vi "Configure Multi Eval Meas Limit Emission Mask Test Tolerance.vi"(7 "Tolerance 30-40 (3.46)":dbl=3.46 format="%^.3e", 8 "error in (no error)":errorcluster, 9 "Tolerance 23-30 (3.21)":dbl=3.21 format="%^.3e", 10 "Instance (1)":T1=1, 11 "VISA resource name":refnum<visa-resource-name>) -> (0 "error out":errorcluster, 3 "VISA resource name out":refnum<visa-resource-name>)   [LabVIEW 2015, in "Rohde&Schwarz CMXP NR FR2 Measurement.lvlib"]
doc: "Defines the test tolerance for spectrum emission masks, depending on the carrier frequency.\n\nAttribute:\nRSCMXPNRFR2M_ATTR_MULTI_EVAL_MEASUREMENT_LIMIT_EMISSION_MASK_TEST_TOLERANCE\n\nRemote-control command:\nCONFigure:NRMMw:MEAS<i>:MEValuation:LIMit:SEMask:ATTolerance"
uses:
  <instrlib>/Rohde&Schwarz CMXP NR FR2 Measurement/Rohde&Schwarz CMXP NR FR2 Measurement.lvlib
  <instrlib>/Rohde&Schwarz CMXP NR FR2 Measurement/Private/_Instance.ctl
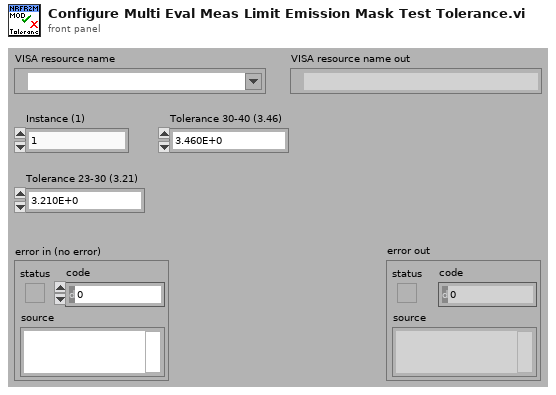
[diagram p1: front panel]
types:
  T1 = typedef "Rohde&Schwarz CMXP NR FR2 Measurement.lvlib/_Instance.ctl" = i32
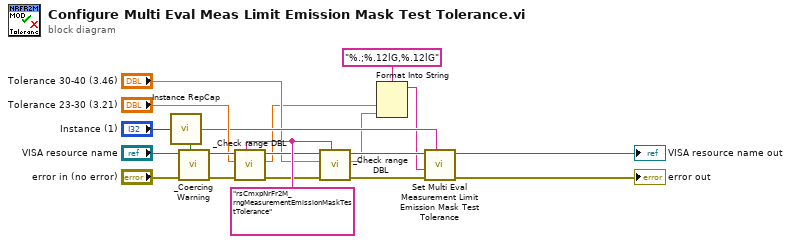
[diagram p0: block diagram]
diagram:
  w17 = "rsCmxpNrFr2M_rngMeasurementEmissionMaskTestTolerance"
  n1 = call <instrlib>:"Instance RepCap.vi"("Instance In"="Instance (1)") -> ("In Range?"=w18:bool, "RepCap Identifier Out"=w8:string)  [unwired: 1 in]
  n2 = call <instrlib>:"_Coercing Warning.vi"("In Range?"=w18, "error in (no error)"="error in (no error)", "VISA resource name"="VISA resource name") -> ("error out"=w15:errorcluster, "VISA resource name out"=w16:refnum<visa-resource-name>)  [unwired: 7 in]
  n3 = call <instrlib>:"_Check range DBL.vi"("Range Table Identifier"=w17, "error in (no error)"=w15, "DBL Value In"="Tolerance 23-30 (3.21)", "VISA resource name"=w16) -> ("error out"=w12:errorcluster, "DBL Value Out"=w4:dbl, "VISA resource name out"=w13:refnum<visa-resource-name>)  [unwired: 5 in]
  n4 = call <instrlib>:"_Check range DBL.vi"("Range Table Identifier"=w17, "error in (no error)"=w12, "DBL Value In"="Tolerance 30-40 (3.46)", "VISA resource name"=w13) -> ("error out"=w9:errorcluster, "DBL Value Out"=w3:dbl, "VISA resource name out"=w10:refnum<visa-resource-name>)  [unwired: 5 in]
  n5 = Format Into String(format string="%.;%.12lG,%.12lG", w4, w3) -> (resulting string=w1:string)  [unwired: 2 in, 1 out]
  n6 = call "Set Multi Eval Measurement Limit Emission Mask Test Tolerance"("Repeated Capabilities"=w8, "error in (no error)"=w9, "Multi Eval Measurement Limit Emission Mask Test Tolerance ()"=w1, "instrument handle"=w10) -> ("error out"=→"error out":errorcluster, "instrument handle out"=→"VISA resource name out":refnum<visa-resource-name>)  [unwired: 6 in]
